vi "Next_Temp_Field.vi"(6 "Numeric in":i32, 7 "Field and Temp Range":T1={"VISA (Magnet)"="COM4", "Fields(T)"=[], "Temps(K)"=[], "VISA (Temp) "="COM1", "Port number (3364)"=3364}, 8 "error in (no error)":errorcluster, 9 "TempQ in":refnum<queue>, 10 "MagQ in":refnum<queue>, 11 "Queue in":refnum<queue>) -> (0 "error out":errorcluster, 1 "TempQ out":refnum<queue>, 2 "MagQ out":refnum<queue>, 3 "Queue out":refnum<queue>, 5 "Numeric out":i32)   [LabVIEW 2025]
uses:
  Mag & Temp STM/CTLS/Sweeper.ctl
  Mag & Temp STM/CTLS/PSU Status.ctl
  Downloads/OneDrive_2025-09-03/Instrument Controls/Temp Cntrl.ctl
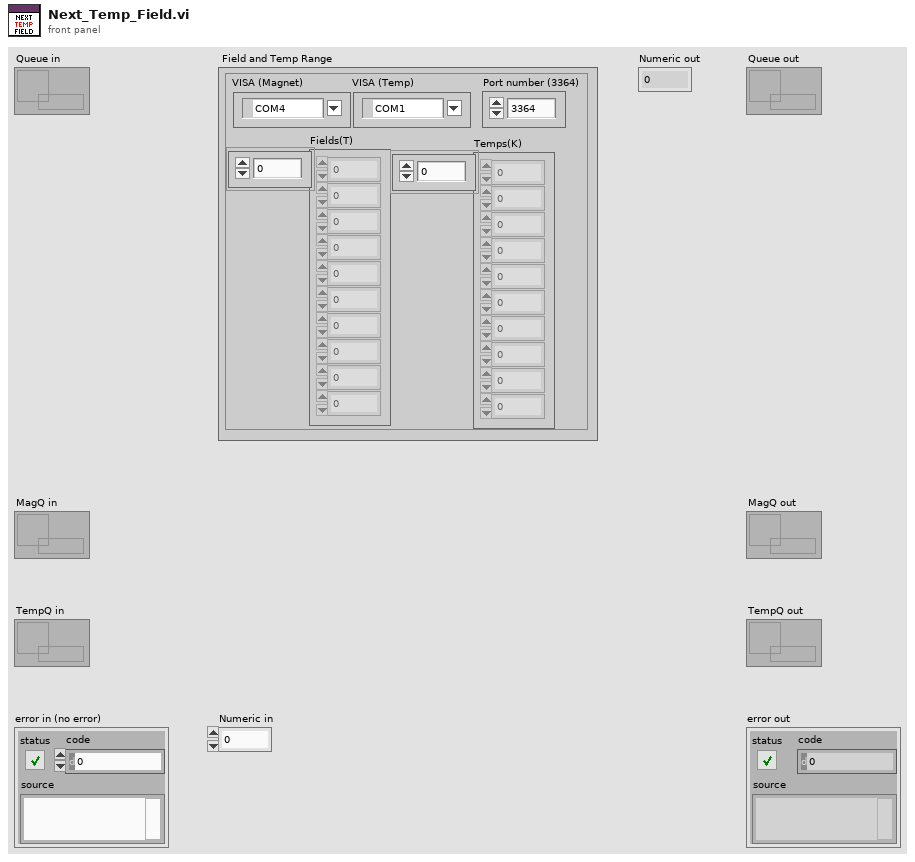
[diagram p1: front panel]
types:
  T1 = cluster{"VISA (Magnet)":refnum<visa-resource-name>, "Fields(T)":dbl[], "Temps(K)":dbl[], "VISA (Temp) ":refnum<visa-resource-name>, "Port number (3364)":u32}
  T2 = enum16{"NO CHANGE", "SET TEMP & FIELD", "SWEEP IDLE", "NEXT TEMP & FIELD", "SWEEP DONE"}
  T3 = typedef "Sweeper.ctl" = cluster{"Temps(K)":dbl[], "Fields(T)":dbl[], "Sweep States":enum16{"1. Idle", "2. Start", "3. Apply_Config", "4. Run_Point_Step", "5. Wait ACK", "6. Next Field", "7. Next Temp", "8. Stop"}, "PointStep":enum16{"1. Scan_1", "2. DC_SF_1", "3. DC_BS_1", "4. Bias", "5. Scan_2", "6. DC_SF_2", "7. DC_BS_2", "8. Done"}, "Current Field":dbl, "Current Temp":dbl, "Expected_ACK":enum16{"1. None", "2. TempStable", "3. FieldStable", "4. ConfigApplied", "5. ScanDone", "6. BiasDone", "7. DriftDone (SF)", "8. DrifDone (BS)", "9. Done"}, "ACK":enum16{"1. None", "2. TempStable", "3. FieldStable", "4. ConfigApplied", "5. ScanDone", "6. BiasDone", "7. DriftDone (SF)", "8. DrifDone (BS)", "9. Done"}, "AfterAckStep":enum16{"1. Idle", "2. Start", "3. Apply_Config", "4. Run_Point_Step", "5. Wait ACK", "6. Next Field", "7. Next Temp", "8. Stop"}, "Current Index Field":i32, "Current Index Temp":i32, "ACK Structure ":enum16{"Inner", "Outer"}}
  T4 = typedef "Temp Cntrl.ctl" = cluster{"Range (0:Off)":u16, "Manual Output (0.00 %)":dbl, "Rate (D) (0.0 %)":dbl, "Reset (I) (20.0)":dbl, "Gain (P) (50.0)":dbl, "Power Up Enable (F: Disable)":bool, "Max User Current (2.000)":dbl, "Heater Resistance (1:25 Ohms)":u16, "Max Current (0:User Specified)":u16, "Heater Out Display (1:Current)":u16, "Mode (0:Off)":u16, "Input (0:None)":u16, "Target Temp (K)":dbl, "Serial Configuration":cluster{"Baud Rate":u32, "Parity":u16, "Data Bits":u16, "Stop Bits":u16, "Flow Control":u16}, "VISA resource name":refnum<visa-resource-name>, "Configure Control Parameters (0: Configure)":u16, "Enable Setpoint (F:Disable)":bool, "Input (0:A)":u16, "Data Source (0:Kelvin)":u16, "Output's Control Loop (1:1)":u16, "STND DEV Threshold ":dbl, "Mean Tolerance ":dbl, "Current State":enum16{"1. INIT TEMP", "2. TC ON", "3. POLL_TEMPS", "4. TEMP_STAB", "5. TC IDLE", "6. APPLY NEXT TEMP", "7. TC OFF (Reset)"}}
  T5 = enum16{"1. INIT TEMP", "2. TC ON", "3. POLL_TEMPS", "4. TEMP_STAB", "5. TC IDLE", "6. APPLY NEXT TEMP", "7. TC OFF (Reset)"}
  T6 = enum16{"1. INIT MAG", "2. MAG ON", "3. MAG_STAB", "4. MAG IDLE", "5. PREP NEXT FIELD", "6. APPLY NEXT FIELD", "7. PREP OFF", "8. MAG OFF (Reset)"}
  T7 = typedef "PSU Status.ctl" = cluster{"Ramp Target":enum16{"ZERO", "MID", "MAX"}, "Pause":bool, "Switch Heater":bool, "Persistent Field":dbl, "Persistent Current":dbl, "Tesla":bool, "Output (T)":dbl, "Output (A)":dbl, "X Trip":enum16{"DISABLED", "ENABLED", "ACTIVE"}, "Ramp Rate (A/s)":dbl, "V Limit (V)":dbl, "Heater Voltage":dbl, "MAX Setpoint (A)":dbl, "MAX Setpoint (T)":dbl, "MID Setpoint (A)":dbl, "MID Setpoint (T)":dbl, "Lock":bool, "Field Constant":dbl, "Remote":bool, "Direction":enum16{"POSITIVE", "NEGATIVE", "OPEN", "UNIPOLAR"}, "Helium Level":u16, "Quench !":bool, "Voltage":dbl, "V Limit !":bool, "Ramping":bool, "At Target":bool, "Trip Field":dbl, "Trip Current":dbl, "Current State":enum16{"1. INIT MAG", "2. MAG ON", "3. MAG_STAB", "4. MAG IDLE", "5. MAG OFF (Reset)"}, "MAG Reference":refnum<visa-resource-name>}
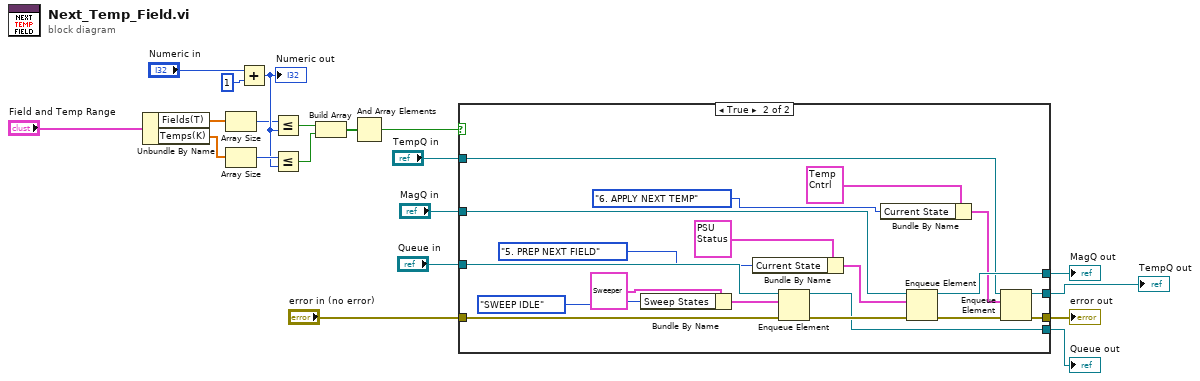
[diagram p0: block diagram]
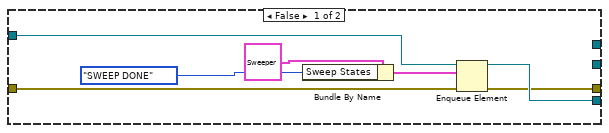
[diagram p2: hidden frame]
diagram:
  n1 = Unbundle By Name("Field and Temp Range") -> ("Fields(T)"=w7:dbl[], "Temps(K)"=w8:dbl[])
  n2 = Array Size(array=w7) -> (size(s)=w6:i32)
  n3 = Array Size(array=w8) -> (size(s)=w10:i32)
  n4 = Add(x="Numeric in", y=1) -> (x+y=w9:i32)
  "Numeric out" <- w9
  n5 = Less Or Equal?(x=w6, y=w9) -> (x <= y?=w11:bool)
  n6 = Less Or Equal?(x=w10, y=w9) -> (x <= y?=w12:bool)
  n7 = Build Array(w11, w12) -> (w13:bool[])
  n8 = And Array Elements(Boolean array=w13) -> (logical AND=w14:bool)
  n9 = case shown="True" w14 {
    tunnel: "Queue in" -> [w24 w44]
    tunnel: "MagQ in" -> [_ w43]
    tunnel: [w23 w37] -> w17
    tunnel: [_ w36] -> w18
    tunnel: "TempQ in" -> [_ w34]
    tunnel: [w22 w31] -> w19
    tunnel: [_ w30] -> w2
    tunnel: "error in (no error)" -> [w21 w29]
    frame False {
      n10 = Bundle By Name(cluster=T3 {"Temps(K)"=[], "Fields(T)"=[], "Sweep States"=enum."2. Start", "PointStep"=enum."1. Scan_1", "Current Field"=0.0, "Current Temp"=0.0, "Expected_ACK"=enum."1. None", "ACK"=enum."1. None", "AfterAckStep"=enum."1. Idle", "Current Index Field"=-1, "Current Index Temp"=-1, "ACK Structure "=enum."Inner"} ("Temp and Field Range"), "Sweep States"=T2."SWEEP DONE") -> (w26:T3)
      n11 = Enqueue Element(queue=w24, element=w26, error in (no error)=w21) -> (queue out=w23:refnum<queue>, error out=w22:errorcluster)  [unwired: 1 in, 1 out]
    }
    frame True {
      n12 = Bundle By Name(cluster=T3 {"Temps(K)"=[], "Fields(T)"=[], "Sweep States"=enum."2. Start", "PointStep"=enum."1. Scan_1", "Current Field"=0.0, "Current Temp"=0.0, "Expected_ACK"=enum."1. None", "ACK"=enum."1. None", "AfterAckStep"=enum."1. Idle", "Current Index Field"=-1, "Current Index Temp"=-1, "ACK Structure "=enum."Inner"} ("Temp and Field Range"), "Sweep States"=T2."SWEEP IDLE") -> (w45:T3)
      n13 = Bundle By Name(cluster=T7 {"Ramp Target"=enum."ZERO", "Pause"=FALSE, "Switch Heater"=FALSE, "Persistent Field"=0.0, "Persistent Current"=0.0, "Tesla"=FALSE, "Output (T)"=0.0, "Output (A)"=0.0, "X Trip"=enum."DISABLED", "Ramp Rate (A/s)"=0.0, "V Limit (V)"=0.0, "Heater Voltage"=0.0, "MAX Setpoint (A)"=0.0, "MAX Setpoint (T)"=0.0, "MID Setpoint (A)"=0.0, "MID Setpoint (T)"=0.0, "Lock"=FALSE, "Field Constant"=0.0, "Remote"=FALSE, "Direction"=enum."POSITIVE", "Helium Level"=0, "Quench !"=FALSE, "Voltage"=0.0, "V Limit !"=FALSE, "Ramping"=FALSE, "At Target"=FALSE, "Trip Field"=0.0, "Trip Current"=0.0, "Current State"=enum."1. INIT MAG", "MAG Reference"="COM4"} ("PSU Status In"), "Current State"=T6."5. PREP NEXT FIELD") -> (w41:T7)
      n14 = Enqueue Element(queue=w44, element=w45, error in (no error)=w29) -> (queue out=w37:refnum<queue>, error out=w38:errorcluster)  [unwired: 1 in, 1 out]
      n15 = Bundle By Name(cluster=T4 {"Range (0:Off)"=0, "Manual Output (0.00 %)"=0.0, "Rate (D) (0.0 %)"=0.0, "Reset (I) (20.0)"=20.0, "Gain (P) (50.0)"=50.0, "Power Up Enable (F: Disable)"=FALSE, "Max User Current (2.000)"=2.0, "Heater Resistance (1:25 Ohms)"=1, "Max Current (0:User Specified)"=0, "Heater Out Display (1:Current)"=1, "Mode (0:Off)"=1, "Input (0:None)"=4, "Target Temp (K)"=5.0, "Serial Configuration"={"Baud Rate"=57600, "Parity"=1, "Data Bits"=7, "Stop Bits"=10, "Flow Control"=0}, "VISA resource name"="", "Configure Control Parameters (0: Configure)"=0, "Enable Setpoint (F:Disable)"=FALSE, "Input (0:A)"=3, "Data Source (0:Kelvin)"=0, "Output's Control Loop (1:1)"=2, "STND DEV Threshold "=0.1, "Mean Tolerance "=0.02, "Current State"=enum."1. INIT TEMP"} ("element"), "Current State"=T5."6. APPLY NEXT TEMP") -> (w33:T4)
      n16 = Enqueue Element(queue=w43, element=w41, error in (no error)=w38) -> (queue out=w36:refnum<queue>, error out=w35:errorcluster)  [unwired: 1 in, 1 out]
      n17 = Enqueue Element(queue=w34, element=w33, error in (no error)=w35) -> (queue out=w30:refnum<queue>, error out=w31:errorcluster)  [unwired: 1 in, 1 out]
    }
  }
  "error out" <- w19
  "MagQ out" <- w18
  "Queue out" <- w17
  "TempQ out" <- w2
